vi "Scout2String.vi"(9 "Scores":T1, 10 "Auto":T2, 11 "Team":T3) -> (1 "String":string, 2 "Match":string, 3 "Team":u16)   [LabVIEW 2013]
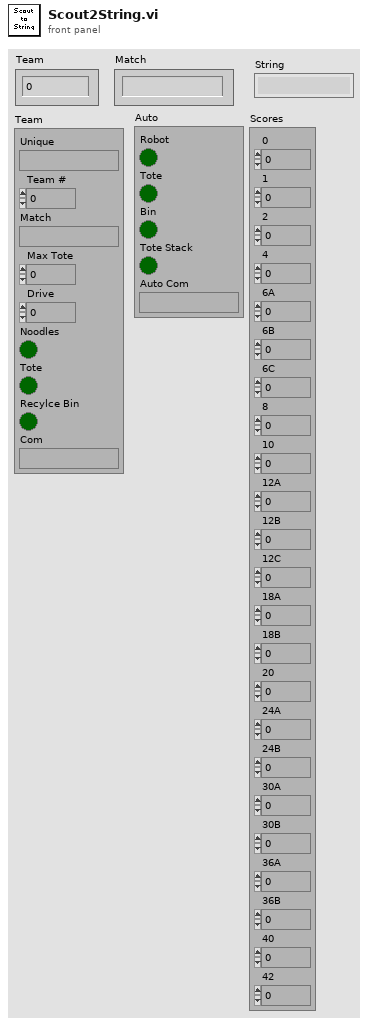
[diagram p1: front panel]
types:
  T1 = cluster{"0":u8, "1":u8, "2":u8, "4":u8, "6A":u8, "6B":u8, "6C":u8, "8":u8, "10":u8, "12A":u8, "12B":u8, "12C":u8, "18A":u8, "18B":u8, "20":u8, "24A":u8, "24B":u8, "30A":u8, "30B":u8, "36A":u8, "36B":u8, "40":u8, "42":u8}
  T2 = cluster{"Robot":bool, "Tote":bool, "Bin":bool, "Tote Stack":bool, "Auto Com":string}
  T3 = cluster{"Unique":string, "Team #":u16, "Match":string, "Max Tote":u8, "Drive":u16, "Noodles":bool, "Tote":bool, "Recylce Bin":bool, "Com":string}
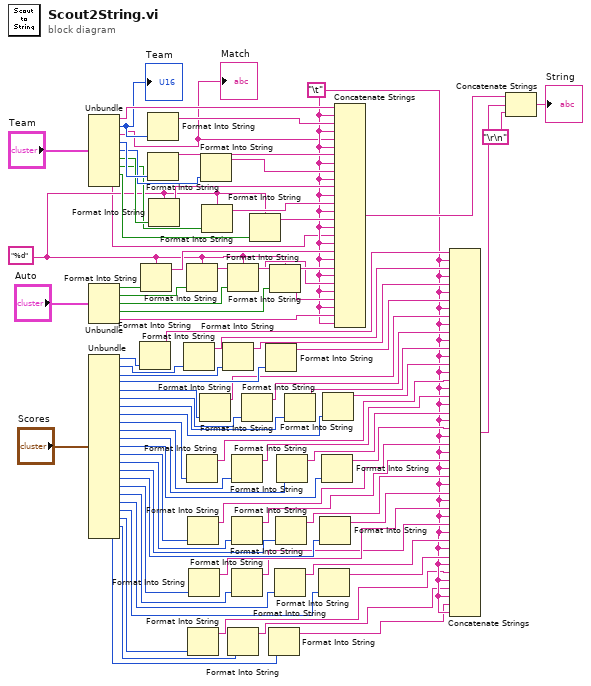
[diagram p0: block diagram]
diagram:
  w6 = "%d" ("format string")
  w13 = "\t"
  n1 = Unbundle("Team") -> ("Unique"=w79:string, "Team #"=w9:u16, "Match"=w8:string, "Max Tote"=w77:u8, "Drive"=w75:u16, "Noodles"=w73:bool, "Tote"=w72:bool, "Recylce Bin"=w71:bool, "Com"=w5:string)
  "Match" <- w8
  "Team" <- w9
  n2 = Unbundle("Auto") -> ("Robot"=w67:bool, "Tote"=w66:bool, "Bin"=w65:bool, "Tote Stack"=w64:bool, "Auto Com"=w59:string)
  n3 = Unbundle("Scores") -> ("0"=w58:u8, "1"=w57:u8, "2"=w56:u8, "4"=w55:u8, "6A"=w49:u8, "6B"=w48:u8, "6C"=w47:u8, "8"=w42:u8, "10"=w40:u8, "12A"=w39:u8, "12B"=w38:u8, "12C"=w37:u8, "18A"=w36:u8, "18B"=w35:u8, "20"=w34:u8, "24A"=w33:u8, "24B"=w24:u8, "30A"=w23:u8, "30B"=w22:u8, "36A"=w21:u8, "36B"=w20:u8, "40"=w19:u8, "42"=w18:u8)
  n4 = Format Into String(w58) -> (resulting string=w53:string)  [unwired: 3 in, 1 out]
  n5 = Format Into String(format string=w6, w67) -> (resulting string=w63:string)  [unwired: 2 in, 1 out]
  n6 = Format Into String(w9) -> (resulting string=w78:string)  [unwired: 3 in, 1 out]
  n7 = Format Into String(w77) -> (resulting string=w76:string)  [unwired: 3 in, 1 out]
  n8 = Format Into String(format string=w6, w73) -> (resulting string=w70:string)  [unwired: 2 in, 1 out]
  n9 = Format Into String(w57) -> (resulting string=w51:string)  [unwired: 3 in, 1 out]
  n10 = Format Into String(format string=w6, w66) -> (resulting string=w62:string)  [unwired: 2 in, 1 out]
  n11 = Format Into String(w40) -> (resulting string=w32:string)  [unwired: 3 in, 1 out]
  n12 = Format Into String(w36) -> (resulting string=w28:string)  [unwired: 3 in, 1 out]
  n13 = Format Into String(w20) -> (resulting string=w12:string)  [unwired: 3 in, 1 out]
  n14 = Format Into String(w24) -> (resulting string=w17:string)  [unwired: 3 in, 1 out]
  n15 = Format Into String(w49) -> (resulting string=w46:string)  [unwired: 3 in, 1 out]
  n16 = Format Into String(w75) -> (resulting string=w74:string)  [unwired: 3 in, 1 out]
  n17 = Format Into String(format string=w6, w72) -> (resulting string=w69:string)  [unwired: 2 in, 1 out]
  n18 = Format Into String(w56) -> (resulting string=w50:string)  [unwired: 3 in, 1 out]
  n19 = Format Into String(format string=w6, w65) -> (resulting string=w61:string)  [unwired: 2 in, 1 out]
  n20 = Format Into String(w19) -> (resulting string=w11:string)  [unwired: 3 in, 1 out]
  n21 = Format Into String(w39) -> (resulting string=w31:string)  [unwired: 3 in, 1 out]
  n22 = Format Into String(w35) -> (resulting string=w27:string)  [unwired: 3 in, 1 out]
  n23 = Format Into String(w23) -> (resulting string=w16:string)  [unwired: 3 in, 1 out]
  n24 = Format Into String(w48) -> (resulting string=w45:string)  [unwired: 3 in, 1 out]
  n25 = Format Into String(format string=w6, w71) -> (resulting string=w68:string)  [unwired: 2 in, 1 out]
  n26 = Format Into String(w55) -> (resulting string=w52:string)  [unwired: 3 in, 1 out]
  n27 = Format Into String(w18) -> (resulting string=w10:string)  [unwired: 3 in, 1 out]
  n28 = Format Into String(format string=w6, w64) -> (resulting string=w60:string)  [unwired: 2 in, 1 out]
  n29 = Format Into String(w22) -> (resulting string=w15:string)  [unwired: 3 in, 1 out]
  n30 = Format Into String(w34) -> (resulting string=w26:string)  [unwired: 3 in, 1 out]
  n31 = Format Into String(w38) -> (resulting string=w30:string)  [unwired: 3 in, 1 out]
  n32 = Format Into String(w47) -> (resulting string=w44:string)  [unwired: 3 in, 1 out]
  n33 = Format Into String(w21) -> (resulting string=w14:string)  [unwired: 3 in, 1 out]
  n34 = Format Into String(w33) -> (resulting string=w25:string)  [unwired: 3 in, 1 out]
  n35 = Format Into String(w37) -> (resulting string=w29:string)  [unwired: 3 in, 1 out]
  n36 = Format Into String(w42) -> (resulting string=w43:string)  [unwired: 3 in, 1 out]
  n37 = Concatenate Strings(w79, w13, w78, w13, w8, w13, w76, w13, w74, w13, w70, w13, w69, w13, w68, w13, w5, w13, w63, w13, w62, w13, w61, w13, w60, w13, w59, w13) -> (w54:string)
  n38 = Concatenate Strings(w53, w13, w51, w13, w50, w13, w52, w13, w46, w13, w45, w13, w44, w13, w43, w13, w32, w13, w31, w13, w30, w13, w29, w13, w28, w13, w27, w13, w26, w13, w25, w13, w17, w13, w16, w13, w15, w13, w14, w13, w12, w13, w11, w13, w10, w13) -> (w41:string)
  n39 = Concatenate Strings(w54, w41, "\r\n") -> (→"String":string)
